vi "Is Concrete Class.vi"(0 "SA Path Group in":refnum<class "SA Path Group.lvclass">, 11 "error in":errorcluster) -> (4 "SA Path Group out":refnum<class "SA Path Group.lvclass">, 6 "Is Concrete Class?":bool, 15 "error out":errorcluster)   [LabVIEW 2023, in "RFFixtureCharact.RMM.lvlib" / "SA Path Group.lvclass"]
uses:
  SA Path Group.lvclass
  SA Path Group.lvclass/SA Path Group.ctl
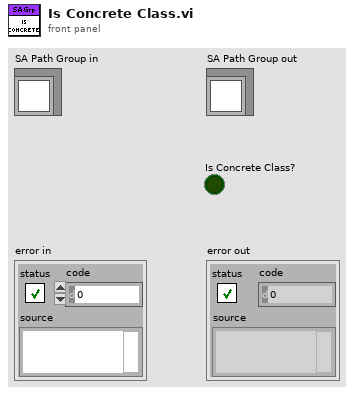
[diagram p1: front panel]
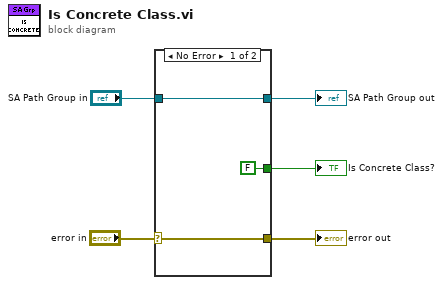
[diagram p0: block diagram]
diagram:
  n1 = case shown="No Error" "error in" {
    selector: "error in" -> [w7 w10]
    tunnel: [FALSE ("Is Concrete Class?") _] -> w1
    tunnel: [w7 w10] -> w4
    tunnel: [w6 w9] -> w3
    tunnel: "SA Path Group in" -> [w6 w9]
    frame No Error {
    }
    frame Error {
    }
  }
  "error out" <- w4
  "SA Path Group out" <- w3
  "Is Concrete Class?" <- w1
